vi "Create Variable File.vi"() -> ()   [LabVIEW 2012]
uses:
  <resource>/objmgr/ni.var.rc
  <vilib>/Utility/VariantDataType/VariantType.lvlib
panel:
  in  "Write?":bool
  in  "Shared Variable File Path":path
  in  "Shared Variable Library Name":string="Shared Variable Test Library"
  in  "IP Address":string="localhost"
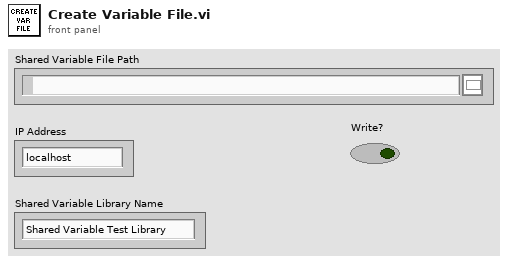
[diagram p1: front panel]
types:
  T1 = enum16{"open", "replace", "create", "open or create", "replace or create", "replace or create with confirmation"}
  T2 = typedef "VariantType.lvlib/Type.ctl" = enum8{"Invalid Type", "Void", "I8", "I16", "I32", "I64", "U8", "U16", "U32", "U64", "Single Float", "Double Float", "Extended Float", "Single Complex", "Double Complex", "Extended Complex", "Enum U8", "Enum U16", "Enum U32", "Enum U64", "Single Float With Unit", "Double Float With Unit", "Extended Float With Unit", "Single Complex with Unit", "Double Complex with Unit", "Extended Complex with Unit", "Boolean", "String", "Path", "Picture", "Tag", "Array", "Cluster", "Variant", "LV Variant", "Waveform", "Timestamp", "Digital Waveform", "Digital Data", "ExpressData", "Refnum", "External Data", "VI", "Poly VI", "LabVIEW Class Instance", "Fixed Point"}
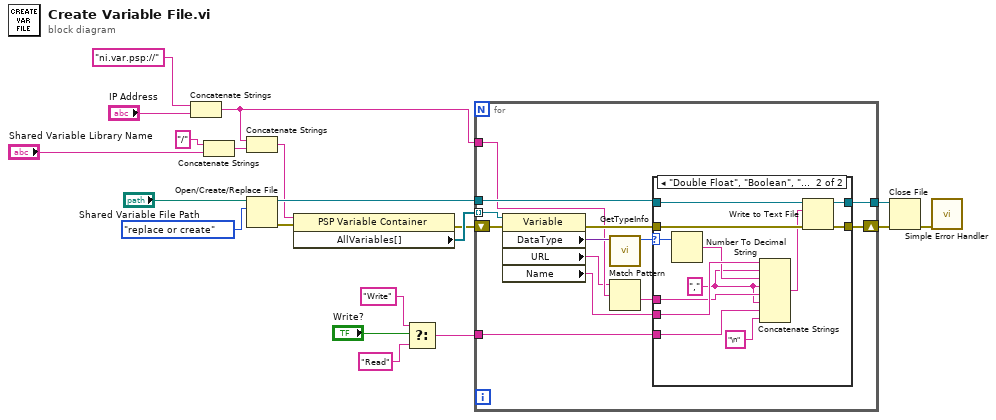
[diagram p0: block diagram]
diagram:
  n1 = Concatenate Strings("ni.var.psp://" ("PSP URL"), "IP Address") -> (w5:string)
  n2 = Concatenate Strings("/" ("string"), "Shared Variable Library Name") -> (w7:string)
  n3 = Concatenate Strings(w5, w7) -> (w6:string)
  n4 = Open/Create/Replace File(file path (use dialog)="Shared Variable File Path", operation (0:open)=T1."replace or create") -> (refnum out=w13:refnum<file>, error out=w14:errorcluster)  [unwired: 4 in, 1 out]
  n5 = property class="PSP Variable Container"(reference=w6, error in=w14) -> (error out=w19:errorcluster, "AllVariables[]"=w20:refnum<k21>[])  [unwired: 1 out]
  n6 = Select(t="Write", s="Write?", f="Read") -> (s? t:f=w3:string)
  n7 = for {
    tunnel: w20 -> [w32] mode=indexing
    shift-right: [w26] -> w11
    shift-left: w19 -> [w33]
    tunnel: w5 -> [w24]
    tunnel: w13 -> [w28]
    tunnel: [w25] -> w12
    tunnel: w3 -> [w21]
    n8 = property class="Variable"(reference=w32, error in=w33) -> (error out=w27:errorcluster, "DataType"=w31:variant, "URL"=w23:string, "Name"=w29:string)  [unwired: 1 out]
    n9 = call <vilib>:"GetTypeInfo.vi"("Variant"=w31) -> ("Type Enum"=w30:T2)  [unwired: 6 in, 4 out]
    n10 = Match Pattern(string=w23, regular expression=w24) -> (after substring=w22:string)  [unwired: 1 in, 3 out]
    n11 = case shown="\"Double Float\", \"Boolean\", \"String\"" w30 {
      selector: w30 -> [_ w44]
      tunnel: w29 -> [_ w43]
      tunnel: w28 -> [w35 w47]
      tunnel: w27 -> [w34 w46]
      tunnel: [w34 w45] -> w26
      tunnel: [w35 w40] -> w25
      tunnel: w22 -> [_ w38]
      tunnel: w21 -> [_ w36]
      frame Default {
      }
      frame "Double Float", "Boolean", "String" {
        w37 = "," ("string")
        n12 = Number To Decimal String(number=w44) -> (decimal integer string=w42:string)  [unwired: 1 in]
        n13 = Concatenate Strings(w43, w37, w42, w37, w38, w37, w36, "\n" ("string")) -> (w41:string)
        n14 = Write to Text File(file (use dialog)=w47, text=w41, error in=w46) -> (refnum out=w40:refnum<file>, error out=w45:errorcluster)  [unwired: 1 in, 1 out]
      }
    }
  }
  n15 = Close File(refnum=w12, error in=w11) -> (error out=w10:errorcluster)  [unwired: 1 out]
  n16 = call <vilib>:"Simple Error Handler.vi"("error in (no error)"=w10) -> ()  [unwired: 4 in, 5 out]
